vi "Build Modbus Wfm Header.vi"(8 "error in (no error)":errorcluster, 11 "DAQ Task in":refnum<class "DAQ Task.lvclass">) -> (0 "error out":errorcluster, 2 "Wfm Header":T1, 3 "DAQ Task out":refnum<class "DAQ Task.lvclass">)   [LabVIEW 2018, in "Data Acquisition.lvlib" / "DAQ Task.lvclass"]
uses:
  DAQ Task.lvclass
  Common/Controls/Waveform Header.ctl
  DAQ Task.lvclass/DAQ Task.ctl
  Measurements/Class Channel/Read ToModBus.vi
  Measurements/Class Channel/Read ChanName.vi
  Measurements/Class Channel/Read Unit_EU.vi
  Measurements/Class Channel/Channel.lvclass
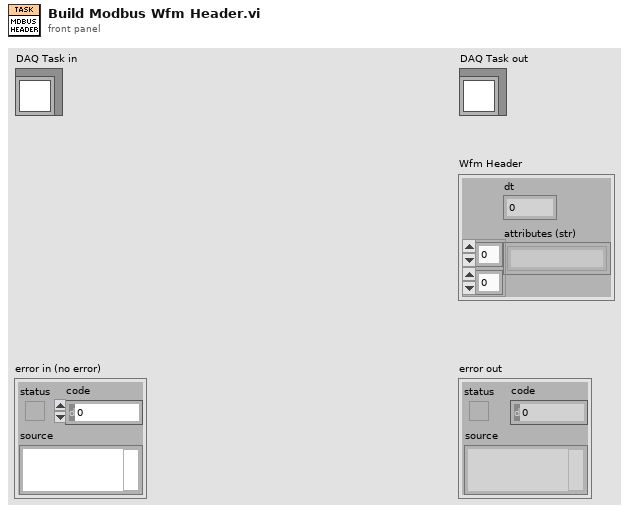
[diagram p1: front panel]
types:
  T1 = typedef "Waveform Header.ctl" = cluster{"dt":dbl, "attributes (str)":string[][]}
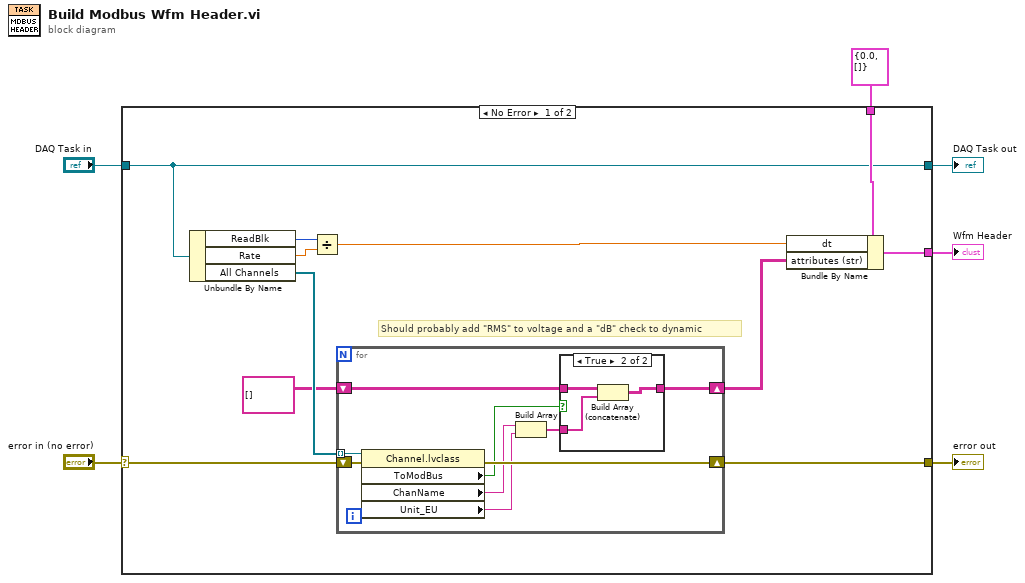
[diagram p0: block diagram]
diagram:
  n1 = case shown="No Error" "error in (no error)" {
    selector: "error in (no error)" -> [w10 w33]
    tunnel: [w9 w33] -> w5
    tunnel: [w15 w32] -> w3
    tunnel: "DAQ Task in" -> [w15 w32]
    tunnel: T1 {"dt"=0.0, "attributes (str)"=[]} ("Wfm Header") -> [w17 w31]
    tunnel: [w16 w31] -> w1
    frame No Error {
      # "Should probably add \"RMS\" to voltage and a \"dB\" check to dynamic"
      n2 = Unbundle By Name(w15) -> ("ReadBlk"=w14:i32, "Rate"=w13:dbl, "All Channels"=w11:refnum<class "Channel.lvclass">[])
      n3 = Divide(x=w14, y=w13) -> (x/y=w12:dbl)
      n4 = for {
        tunnel: w11 -> [w26] mode=indexing
        shift-right: [w24] -> w9
        shift-left: w10 -> [w25]
        shift-right: [w18] -> w7
        shift-left: string[][] [] -> [w21]
        n5 = property class="Channel.lvclass"(reference=w26, error in=w25) -> (error out=w24:errorcluster, "ToModBus"=w20:bool, "ChanName"=w22:string, "Unit_EU"=w23:string)  [unwired: 1 out]
        n6 = Build Array(w22, w23) -> (w19:string[])
        n7 = case shown="True" w20 {
          tunnel: w21 -> [w27 w30]
          tunnel: w19 -> [_ w29]
          tunnel: [w27 w28] -> w18
          frame False {
          }
          frame True {
            n8 = Build Array (concatenate)(w30, w29) -> (w28:string[][])
          }
        }
      }
      n9 = Bundle By Name(cluster=w17, "dt"=w12, "attributes (str)"=w7) -> (w16:T1)
    }
    frame Error {
    }
  }
  "error out" <- w5
  "DAQ Task out" <- w3
  "Wfm Header" <- w1
